vi "Mean.vi"   [LabVIEW 2012, in "NI_AALBase.lvlib"]
doc: "Computes the <B>mean</B> of the values in the input sequence <B>X</B>. You must manually select the polymorphic instance you want to use."
uses:
  NI_AALBase.lvlib
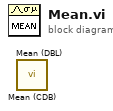
[diagram p0: block diagram]
diagram:
  n1 = call "Mean (CDB).vi"() -> ()  [unwired: 1 in, 2 out]
  n2 = call "Mean (DBL).vi"() -> ()  [unwired: 1 in, 2 out]
